vi "stop_sweep.vi"(8 "error in (no error)":errorcluster, 11 "ScanModeDL090923Scaffold in":refnum<class "ImagingModeDL090923Scaffold.lvclass">) -> (0 "error out":errorcluster, 3 "ScanModeDL090923Scaffold out":refnum<class "ImagingModeDL090923Scaffold.lvclass">)   [LabVIEW 2010, in "ImagingModeDL090923Scaffold.lvclass"]
uses:
  ImagingModeDL090923Scaffold.lvclass
  common/classes/GenericComponent/GenericComponent/class_data.vi
  common/classes/ErrorController/ErrorController/class_data.vi
  ExperimentController/GenericExperimentController/GenericExperimentController/trigger_enum.ctl
  ExperimentController/GenericExperimentController/GenericExperimentController/GenericExperimentController.lvclass
  common/classes/ErrorController/ErrorController/ErrorController.lvclass
  common/classes/GenericComponent/GenericComponent/GenericComponent.lvclass
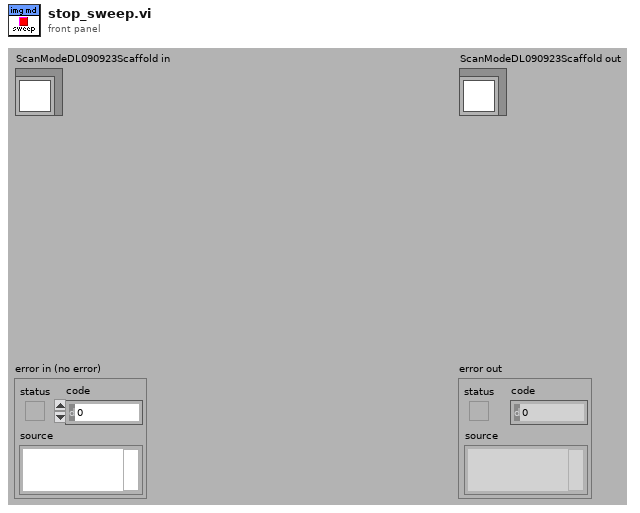
[diagram p1: front panel]
types:
  T1 = typedef "GenericExperimentController.lvclass/trigger_enum.ctl" = enum16{"NULL", "proceed", "prepare"}
  T2 = typedef "GenericToplevelComponent.lvclass/common_trigger_enum.ctl" = enum16{"NULL", "initialise", "terminate", "fetch command", "fetch data", "attach observer", "register as observer", "detach observer", "acknowledge", "start", "stop", "sweep started", "sweep finished", "experiment started", "experiment stopped"}
  T3 = typedef "run_mode_enum.ctl" = enum16{"focus mode", "single sweep mode", "experiment mode"}
  T4 = typedef "main_trigger_enum.ctl" = enum16{"NULL", "initialise", "terminate", "start", "stop", "change objective", "change experimentController", "change imagingMode", "save notebook", "started saving", "finished saving", "expCtr ready", "expCtr missing", "imgMd ready", "imgMd missing", "scanHd ready", "scanHd missing", "DAQ ready", "DAQ missing", "imgAsm ready", "imgAsm missing", "dataColl ready", "dataColl missing", "display ready", "display missing", "analysr ready", "analysr missing", "instrmnt ready", "instrmnt missing", "stimltr ready", "stimltr missing", "stage ready", "stage missing"}
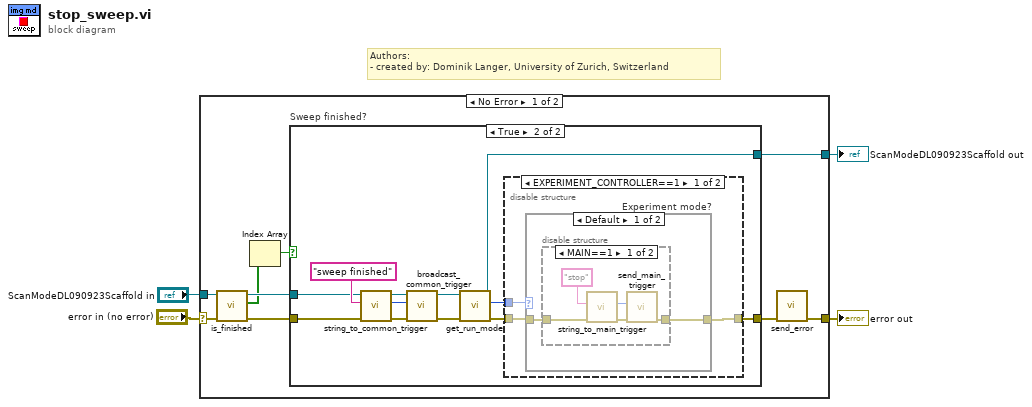
[diagram p0: block diagram]
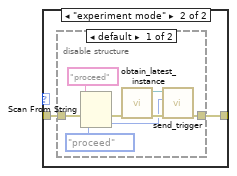
[diagram p4: hidden frame]
diagram:
  # "Authors: \n- created by: Dominik Langer, University of Zurich, Switzerland"
  n1 = case shown="No Error" "error in (no error)" {
    selector: "error in (no error)" -> [w10 w52]
    tunnel: [w13 w52] -> w3
    tunnel: [w11 w51] -> w1
    tunnel: "ScanModeDL090923Scaffold in" -> [w8 w51]
    frame No Error {
      n2 = call-dynamic "is_finished.vi"("error in (no error)"=w10, "ImagingModeDL090923Scaffold in"=w8) -> ("error out"=w9:errorcluster, "finished?"=w6:bool[], "ImagingModeDL090923Scaffold out"=w7:refnum<class "ImagingModeDL090923Scaffold.lvclass">)  [unwired: 7 in]
      n3 = Index Array(array=w6) -> (element=w5:bool)  [unwired: 1 in]
      n4 = case "Sweep finished?" shown="True" w5 {
        tunnel: [w14 w25] -> w12
        tunnel: [w15 w24] -> w11
        tunnel: w9 -> [w14 w20]
        tunnel: w7 -> [w15 w19]
        frame False {
        }
        frame True {
          n5 = call-dynamic "string_to_common_trigger.vi"("error in (no error)"=w20, "trigger string"="sweep finished", "GenericToplevelComponent in"=w19) -> ("error out"=w18:errorcluster, "trigger"=w16:T2, "GenericToplevelComponent out"=w17:refnum<class "ImagingModeDL090923Scaffold.lvclass">)  [unwired: 6 in]
          n6 = call-dynamic "broadcast_common_trigger.vi"("error in (no error)"=w18, "trigger"=w16, "GenericToplevelComponent in"=w17) -> ("error out"=w23:errorcluster, "GenericToplevelComponent out"=w22:refnum<class "ImagingModeDL090923Scaffold.lvclass">)  [unwired: 7 in]
          n7 = call "get_run_mode.vi"("error in (no error)"=w23, "GenericPlugin in"=w22) -> ("error out"=w27:errorcluster, "run mode"=w26:T3, "GenericPlugin out"=w24:refnum<class "ImagingModeDL090923Scaffold.lvclass">)  [unwired: 5 in, 2 out]
          n8 = disable-structure shown="EXPERIMENT_CONTROLLER==1" {
            disable-tunnel: w27 -> [w28 w50]
            disable-tunnel: [w30 w50] -> w25
            disable-tunnel: w26 -> [w29 _]
            frame condition #0 {
              n9 = case "Experiment mode?" shown="Default" w29 {
                tunnel: [w32 w39] -> w30
                tunnel: w28 -> [w31 w40]
                frame Default {
                  n10 = disable-structure shown="MAIN==1" {
                    disable-tunnel: [w37 w38] -> w32
                    disable-tunnel: w31 -> [w36 w38]
                    frame condition #0 {
                      n11 = call "string_to_main_trigger.vi"("error in (no error)"=w36, "trigger string"="stop") -> ("error out"=w34:errorcluster, "main trigger"=w35:T4)  [unwired: 8 in]
                      n12 = call "send_main_trigger.vi"("error in (no error)"=w34, "trigger"=w35) -> ("error out"=w37:errorcluster)  [unwired: 9 in]
                    }
                    frame condition #1 (active) {
                    }
                  }
                }
                frame "experiment mode" {
                  n13 = disable-structure shown="default" {
                    disable-tunnel: w40 -> [w44 w49]
                    disable-tunnel: [w48 w49] -> w39
                    frame condition #0 {
                      n14 = Scan From String(input string="proceed", error in=w44, default 1=trigger_enum."proceed" ("trigger")) -> (error out=w43:errorcluster, output 1=w42:T1)  [unwired: 2 in, 2 out]
                      n15 = call "obtain_latest_instance.vi"("error in (no error)"=w43) -> ("error out"=w47:errorcluster, "GenericExperimentController out"=w46:refnum<class "GenericExperimentController.lvclass">)  [unwired: 1 in, 8 out]
                      n16 = call-dynamic "send_trigger.vi"("error in (no error)"=w47, "trigger"=w42, "GenericExperiment in"=w46) -> ("error out"=w48:errorcluster)  [unwired: 8 out]
                    }
                    frame condition #1 (active) {
                    }
                  }
                }
              }
            }
            frame condition #1 (active) {
            }
          }
        }
      }
      n17 = call "send_error.vi"("error in (no error)"=w12) -> ("error out"=w13:errorcluster)  [unwired: 10 in]
    }
    frame Error {
    }
  }
  "error out" <- w3
  "ScanModeDL090923Scaffold out" <- w1
